vi "Block_User_Interaction.vi"(0 "Reference_In":refnum<vi>[](array[refnum]), 11 "Error_In":errorcluster, 13 "Disabled":T1(ring)=enum."Disabled and Grayed Out") -> (4 "Reference_Out":refnum<vi>[](array[refnum]), 15 "Error_Out":errorcluster)   [LabVIEW 2023, in "File_Handler_Library.lvlib"]
doc: "This VI Blocks the user from entering data to controls"
uses:
  File_Handler_Library.lvlib
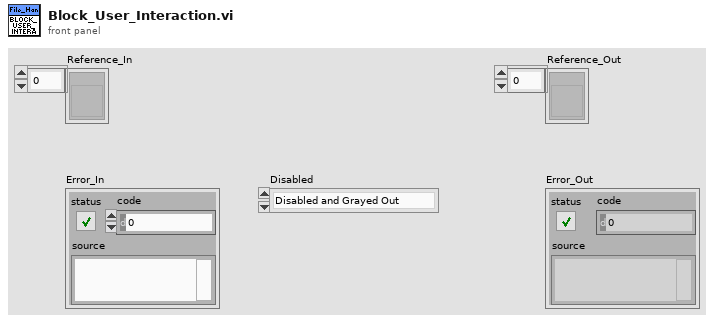
[diagram p1: front panel]
types:
  T1 = enum8{"Enabled", "Disabled", "Disabled and Grayed Out"}
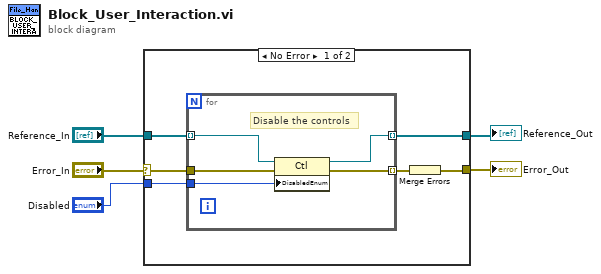
[diagram p0: block diagram]
diagram:
  n1 = case shown="No Error" "Error_In" {
    selector: "Error_In" -> [w8 w18]
    tunnel: "Reference_In" -> [w11 w17]
    tunnel: [w10 w17] -> w4
    tunnel: "Disabled" -> [w9 _]
    tunnel: [w6 w18] -> w1
    frame No Error {
      n2 = for {
        tunnel: [w16] -> w10 mode=indexing
        tunnel: w11 -> [w15] mode=indexing
        tunnel: w9 -> [w14]
        tunnel: w8 -> [w13]
        tunnel: [w12] -> w7 mode=indexing
        # "Disable the controls"
        n3 = property on="Property Node" class="Ctl"(reference=w15, error in=w13, "DisabledEnum"=w14) -> (reference out=w16:refnum<vi>, error out=w12:errorcluster)
      }
      n4 = Merge Errors(w7) -> (w6:errorcluster)
    }
    frame Error {
    }
  }
  "Error_Out" <- w1
  "Reference_Out" <- w4
